vi "ChooseModel.vi"(10 "Array":string[](array[string]), 11 "Information":refnum<vi>) -> (1 "Model":string, 3 "Information":refnum<vi>)   [LabVIEW 2013]
panel:
  in  "OK":bool
  in  "Model":string(combo)
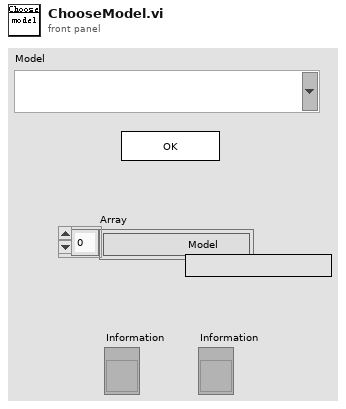
[diagram p1: front panel]
types:
  T1 = typedef "StatusInformation.ctl" = cluster{"FileName:":string, "Barcode(S/N):":string, "TestStep:":string, "TestTime:":string, "Station:":string, "Model:":string, "Line:":string, "Status:":string, "Series:":string, "Reserve:":string}
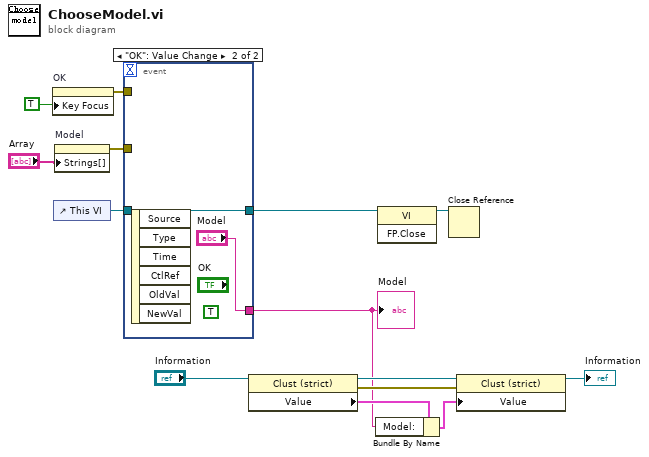
[diagram p0: block diagram]
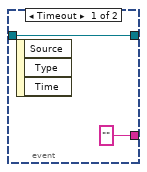
[diagram p2: hidden frame]
diagram:
  n1 = property on="OK" class="Bool"("Key Focus"=TRUE) -> (error out=w2:errorcluster)  [unwired: 2 in, 1 out]
  n2 = control-ref of="This VI"() -> (w12:refnum<vi>)
  n3 = property on="Model" class="CmbBox"("Strings[]"="Array") -> (error out=w10:errorcluster)  [unwired: 2 in, 1 out]
  n4 = event shown="[1] \"OK\": Value Change" {
    selector: _ -> [_ _]
    dyn-events: _ -> [_ _]
    timeout: _ -> [_ _]
    tunnel: ["" ("Model") "Model"] -> w3
    tunnel: w10 -> [_ _]
    tunnel: [w15 w17] -> w13
    tunnel: w12 -> [w15 w17]
    tunnel: w2 -> [_ _]
    event Timeout {
      n5 = event-data() -> ()  [unwired: 1 in, 3 out]
    }
    event "OK": Value Change {
      (unwired) TRUE
      n6 = event-data() -> ()  [unwired: 1 in, 6 out]
    }
  }
  "Model" <- w3
  n7 = property class="Clust (strict)"(reference="Information") -> (reference out=w8:refnum<vi>, error out=w6:errorcluster, "Value"=w7:T1)  [unwired: 1 in]
  n8 = Bundle By Name(cluster=w7, "Model:"=w3) -> (w9:T1)
  n9 = invoke class="VI" method="FP.Close"(reference=w13) -> (reference out=w14:refnum<vi>)  [unwired: 2 in, 2 out]
  n10 = Close Reference(reference=w14) -> ()  [unwired: 1 in, 1 out]
  n11 = property class="Clust (strict)"(reference=w8, error in=w6, "Value"=w9) -> (reference out=→"Information":refnum<vi>)  [unwired: 1 out]
